vi "HEXStringToASCIIString.vi"(7 "Required size (-1)":i32=-1, 8 "error in (no error)":errorcluster, 11 "HEX text in":string) -> (0 "error out":errorcluster, 3 "ASCIIString out":string)   [LabVIEW 2011, in "i3-external-encryption.lvlib"]
doc: "This VI converts an ASCII HEX string (ascii values 0-f) into an array of U8."
uses:
  i3-external-encryption.lvlib
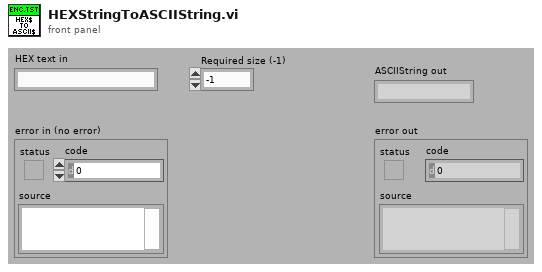
[diagram p1: front panel]
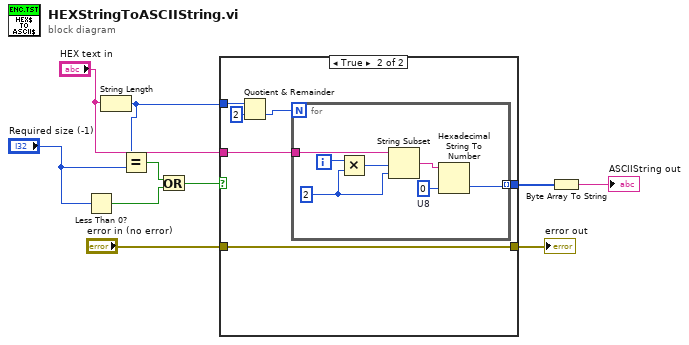
[diagram p0: block diagram]
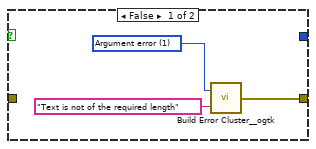
[diagram p2: hidden frame]
diagram:
  n1 = Less Than 0?(x="Required size (-1)") -> (x < 0?=w5:bool)
  n2 = String Length(string="HEX text in") -> (length=w8:i32)
  n3 = Equal?(x=w8, y="Required size (-1)") -> (x = y?=w6:bool)
  n4 = Or(x=w6, y=w5) -> (x .or. y?=w4:bool)
  n5 = case shown="True" w4 {
    tunnel: w8 -> [_ w19]
    tunnel: "HEX text in" -> [_ w16]
    tunnel: [_ w15] -> w9
    tunnel: [w13 w14] -> w3
    tunnel: "error in (no error)" -> [_ w14]
    frame False {
      w12 = 1 items=["No error", "Argument error", "Memory is full", "Out of zone", "End of file", "File already open", "Generic file I/O error", "File not found", "File permission error", "Disk is full", "Duplicate path", "Too many files open", "System feature not enabled", "Resource file not found", "Cannot add resource", "Resource not found", "Image not found", "Image memory error", "Pen does not exist", "Config type invalid", "Config token not found", "Config parse error", "Config memory error", "Bad external code format", "Bad external code offset", "External code not present", "Null window", "Destroy window error", "Null menu", "Print aborted", "Bad print record", "Print driver error", "Windows error during printing", "Memory error during printing", "Print dialog error", "Generic print error", "Invalid device refnum", "Device not found", "Device parameter error", "Device unit error", "Cannot open device", "Device call aborted", "Generic error", "Cancelled by user", "Object ID too low", "Object ID too high", "Object not in heap", "Unknown heap", "Unknown object (invalid DefProc)", "Unknown object (DefProc not in table)", "Message out of range", "Invalid (null) method", "Unknown message", "Manager call not supported", "Bad address", "Network operation in progress", "Network operation timed out", "Connection is busy", "Network attribute not supported", "Network error", "Address in use", "System out of memory", "Connection aborted", "Connection refused", "Not connected", "Already connected", "Connection closed", "Initialization error (interapplication manager)", "Bad occurrence", "Wait on unbound occurrence handler", "Occurrence queue overflow", "Datalog type conflict", "Unused", "Unrecognized type (interapplication manager)", "Memory corrupt", "Failed to make temporary DLL", "Old CIN version", "Drag socket not found", "Failed to load drop-object", "Failed to register OLE object", "Failed to release OLE object", "Format specifier type mismatch", "Unknown format specifier", "Too few format specifiers", "Too many format specifiers", "Scan failed", "Newer CIN version", "Error converting to variant", "Runtime menu error", "Password tampered", "Variant attribute not found", "Incompatible variant data type", "Event data is not available", "Event Store is not present", "Occurrence is not found", "Event Queue is not created", "Event info is not available", "Refnum passed is NULL", "Error retrieving Class GUID", "Error retrieving CoClass GUID", "Error retrieving TypeLib GUID.", "Bad built application magic bytes.", "Specific driver is different from the specific driver associated with the Logical Name.", "There is no session opened to the class driver.", "Max Error", "MAX - Error with config objects", "MAX - Error loading configuration", "MAX - Group not supported"]
      n6 = call <userlib>:"Build Error Cluster__ogtk.vi"("String to Prepend to source (\"\")"="Text is not of the required length" ("String to Prepend to source (\"\")"), "code"=w12) -> ("error out"=w13:errorcluster)
    }
    frame True {
      n7 = Quotient & Remainder(x=w19, y=2) -> (floor(x/y)=w17:i32)  [unwired: 1 out]
      n8 = for {
        N: w17 -> [_]
        tunnel: w16 -> [w26]
        tunnel: [w20] -> w15 mode=indexing
        i -> [w24]
        w21 = u8 0  # U8
        w23 = 2
        n9 = Multiply(x=w24, y=w23) -> (x*y=w25:i32)
        n10 = String Subset(string=w26, offset (0)=w25, length (rest)=w23) -> (substring=w22:string)
        n11 = Hexadecimal String To Number(string=w22, default (0uL)=w21) -> (number=w20:u8)  [unwired: 1 in, 1 out]
      }
    }
  }
  "error out" <- w3
  n12 = Byte Array To String(unsigned byte array=w9) -> (string=→"ASCIIString out":string)
